vi "transmitter.vi"() -> ()   [LabVIEW 2015]
uses:
  <vilib>/addons/Modulation/Digital/General/MT Generate Bits (Galois, PN Order).vi
  <vilib>/addons/Modulation/Digital/Support/Common/Validators/mod_Generate Bits Validate.vi
  <vilib>/addons/Modulation/Analog/support/mod_Set Error Source.vi
  <vilib>/addons/Modulation/Digital/General/MT Generate FSK System Parameters(M).vi
  <vilib>/addons/Modulation/Digital/General/subVIs/mod_Generate Bits PN Sequence.vi
  <vilib>/addons/Modulation/Digital/Support/Common/Validators/mod_Generate Filter Coefficients Validate.vi
  <vilib>/addons/Modulation/Digital/General/subVIs/mod_Generate Filter Coefficients.vi
  <vilib>/addons/Modulation/Analog/MT Upconvert Baseband (Complex).vi
  <instrlib>/niUSRP/niUSRP Write Tx Data (CDB Cluster).vi
  <vilib>/addons/Modulation/niDMT.lvlib
  <vilib>/addons/Modulation/niAMT.lvlib
panel:
  in  "gain":dbl format="%#_6f"
  out "output bit stream":i8[](array[numeric])
  out "upconverted Graph":cluster{"t0":dbl, "dt":dbl, "Y":dbl[]}(graph)
  in  "symbol rate (Hz)":dbl=1.0 format="%.2f"
  in  "symbol phase continuity":enum16{"continuous", "discontinuous"}(ring)
  out "XY Graph":T1(graph)
  in  "total bits (128)":i32=128
  in  "stop button":bool
  in  "pulse shaping filter (none)":T2(ring)
  in  "PN sequence order (9)":i32=9
  in  "modulation type":T3(ring)
  in  "M-FSK (2)":i32=2
  in  "samples per symbol (16)":i32=16
  in  "FSK deviation (Hz)":dbl=150000.0 format="%.2p"
  in  "active antenna":string
  out "coerced carrier frequency":dbl=100000.0 format="%#_6p"
  out "coerced gain":dbl format="%#_6f"
  out "coerced IQ rate":dbl=100000.0 format="%#_6p"
  in  "carrier frequency":dbl=100000.0 format="%#_6p"
  in  "IQ rate":dbl=100000.0 format="%#_6p"
  in  "device names":refnum<k15>
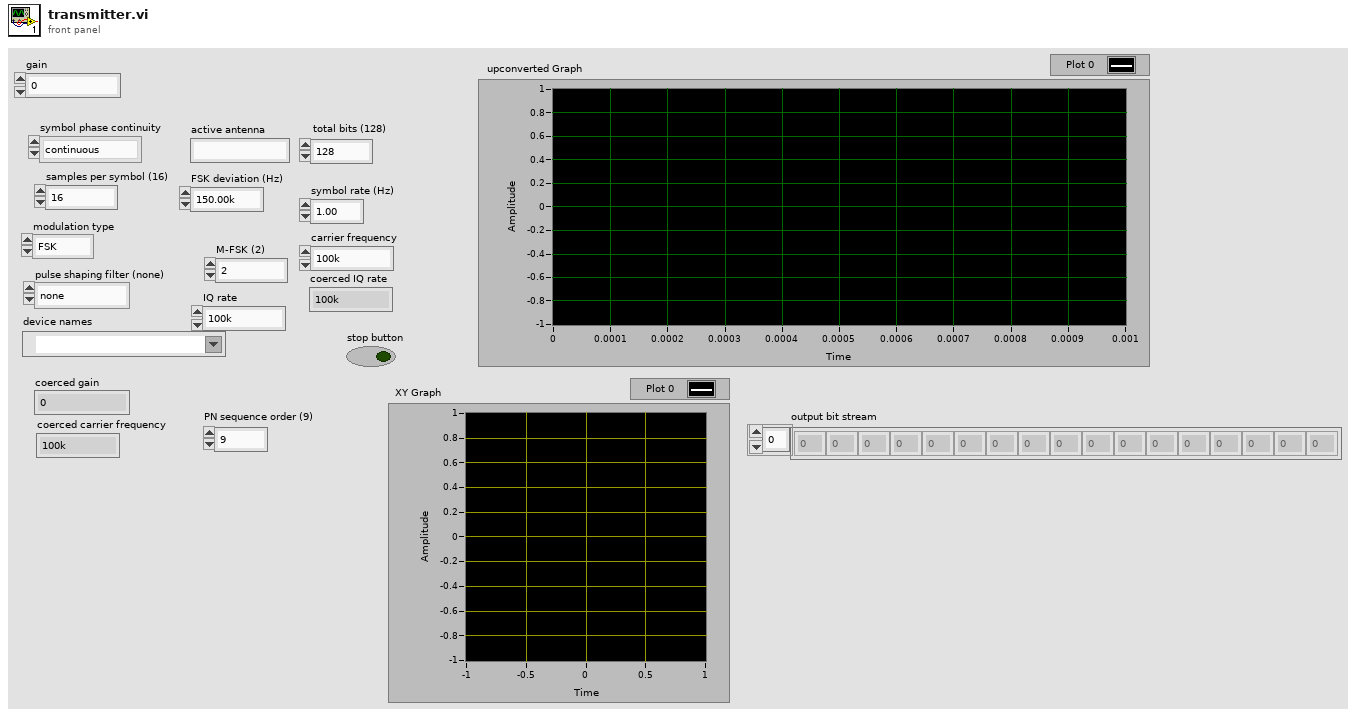
[diagram p1: front panel]
types:
  T1 = cluster{"constellation":dbl[], "oversampled data":dbl[]}[]
  T2 = enum16{"none", "Raised Cosine", "Root Raised Cos", "Gaussian"}
  T3 = enum16{"FSK", "PSK", "QAM", "MSK", "PAM", "ASK", "CPM"}
  T4 = cluster{"samples per symbol (16)":i32, "symbol map":dbl[], "symbol phase continuity":enum16{"continuous", "discontinuous"}}
  T5 = typedef "niAMT.lvlib/Complex Data Waveform.ctl" = cluster{"t0":dbl, "dt":dbl, "Y":cdb[]}
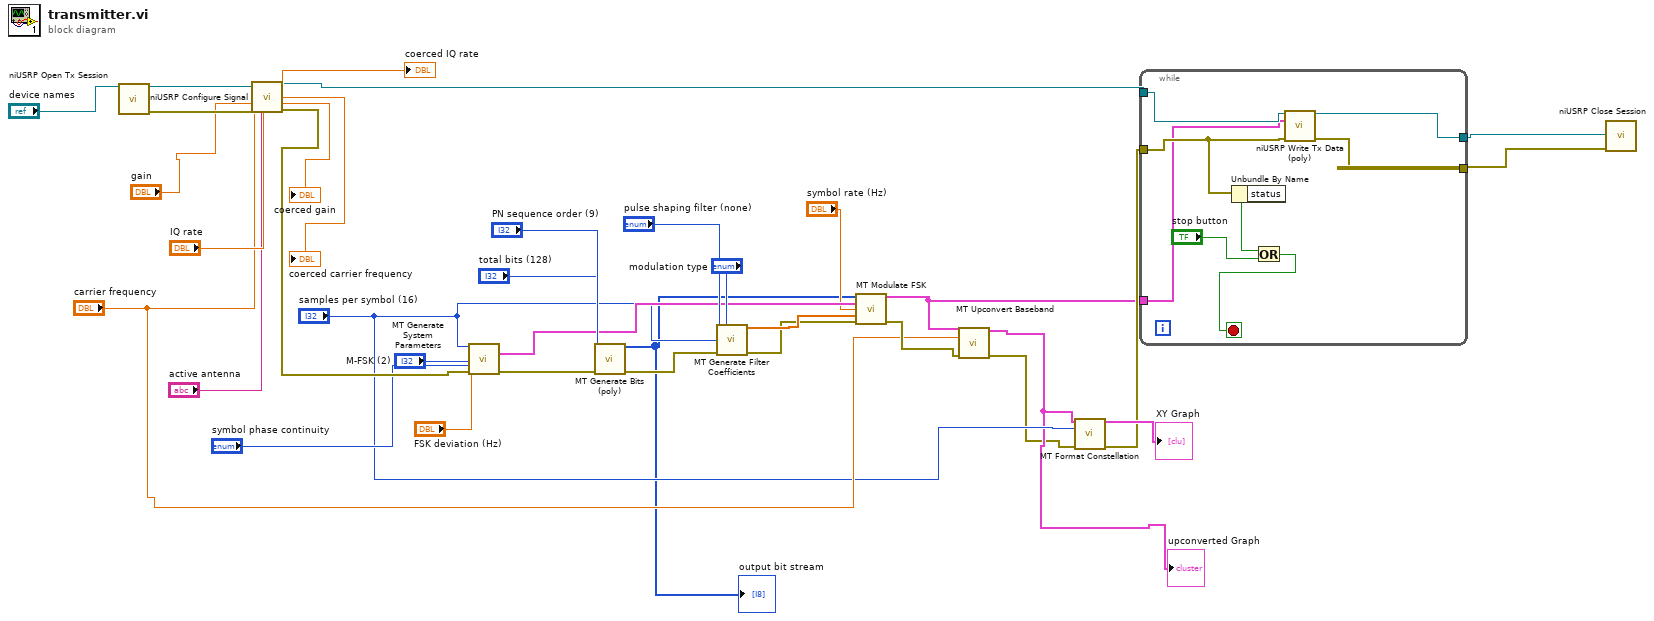
[diagram p0: block diagram]
diagram:
  n1 = call <instrlib>:"niUSRP Open Tx Session.vi"("device names"="device names") -> ("session handle out"=w34:refnum<k15>, "error out"=w32:errorcluster)  [unwired: 13 in]
  n2 = call <instrlib>:"niUSRP Configure Signal.vi"("session handle"=w34, "IQ rate"="IQ rate", "carrier frequency"="carrier frequency", "gain"="gain", "error in (no error)"=w32, "active antenna"="active antenna") -> ("session handle out"=w28:refnum<k15>, "coerced IQ rate"=→"coerced IQ rate":dbl, "coerced carrier frequency"=→"coerced carrier frequency":dbl, "coerced gain"=→"coerced gain":dbl, "error out"=w13:errorcluster)  [unwired: 5 in]
  n3 = call-poly <vilib>:"MT Generate System Parameters.vi"("samples per symbol (16)"="samples per symbol (16)", "M-FSK (2)"="M-FSK (2)", "FSK deviation (Hz)"="FSK deviation (Hz)", "symbol phase continuity"="symbol phase continuity", "error in (no error)"=w13) -> ("FSK system parameters"=w16:T4, "error out"=w23:errorcluster)  [unwired: 8 in, 1 out]
  n4 = call-poly <vilib>:"MT Generate Bits (poly).vi"("total bits (128)"="total bits (128)", "PN sequence order (9)"="PN sequence order (9)", "error in (no error)"=w23) -> ("output bit stream"=w3:i8[], "error out"=w21:errorcluster)  [unwired: 10 in, 1 out]
  "output bit stream" <- w3
  n5 = call <vilib>:"MT Generate Filter Coefficients.vi"("pulse shaping filter (none)"="pulse shaping filter (none)", "modulation type"="modulation type", "matched samples per symbol (16)"="samples per symbol (16)", "error in (no error)"=w21) -> ("pulse shaping filter coefficients"=w22:dbl[], "error out"=w20:errorcluster)  [unwired: 9 in, 1 out]
  n6 = call <vilib>:"MT Modulate FSK.vi"("input bit stream"=w3, "FSK system parameters"=w16, "symbol rate (Hz)"="symbol rate (Hz)", "pulse shaping filter coefficients"=w22, "error in (no error)"=w20) -> ("output complex waveform"=w4:T5, "error out"=w8:errorcluster)  [unwired: 8 in, 1 out]
  n7 = call-poly <vilib>:"MT Upconvert Baseband.vi"("complex waveform"=w4, "carrier frequency (Hz)"="carrier frequency", "error in (no error)"=w8) -> ("upconverted waveform (complex)"=w5:T5, "error out"=w2:errorcluster)  [unwired: 11 in]
  "upconverted Graph" <- w5
  n8 = call <vilib>:"MT Format Constellation.vi"("waveform"=w5, "samples per symbol"="samples per symbol (16)", "error in (no error)"=w2) -> ("constellation graph"=→"XY Graph":T1, "error out"=w12:errorcluster)  [unwired: 11 in]
  n9 = while {
    tunnel: w28 -> [w37]
    tunnel: [w43] -> w26
    tunnel: w12 -> [w38]
    tunnel: [w39] -> w11
    tunnel: w4 -> [w36]
    stop <- w40 stop-if-true
    n10 = Unbundle By Name(w38) -> ("status"=w41:bool)
    n11 = Or(x=w41, y="stop button") -> (x .or. y?=w40:bool)
    n12 = call-poly <instrlib>:"niUSRP Write Tx Data (poly).vi"("session handle"=w37, "data"=w36, "error in (no error)"=w38) -> ("session handle out"=w43:refnum<k15>, "error out"=w39:errorcluster)  [unwired: 11 in]
  }
  n13 = call <instrlib>:"niUSRP Close Session.vi"("session handle"=w26, "error in (no error)"=w11) -> ()  [unwired: 13 in, 1 out]
